vi "top.vi"   [LabVIEW 2009]
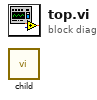
[diagram p0: block diagram]
diagram:
  n1 = call "child.vi"() -> ()  [unwired: 1 in]
